vi "Tree Icons.vi"() -> (1 "not selected":i32, 2 "selected":i32)   [LabVIEW 2021, in "Converter.lvlib"]
uses:
  Converter.lvlib
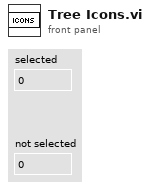
[diagram p1: front panel]
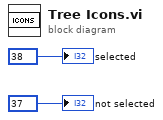
[diagram p0: block diagram]
diagram:
  "selected" <- 38
  "not selected" <- 37
